vi "AS7261_colorimeter.vi"() -> ()   [LabVIEW 2011]
uses:
  <vilib>/Utility/miscctls.llb/LVAnnotationListTypeDef.ctl
  <vilib>/Instr/_visa.llb/VISA Configure Serial Port (Instr).vi
  <vilib>/Analysis/baseanly.llb/A x Vector.vi
  <vilib>/Utility/file.llb/Write To Spreadsheet File (DBL).vi
  <vilib>/Analysis/NI_AALBase.lvlib
panel:
  in  "chrm. adaptation":bool
  in  "OK Button 3":bool
  in  "OK Button 2":bool
  out "count":u16
  out "CTN":string
  out "xy":string
  out "RGB":string
  out "XYZ data":string
  out "XYZ array":dbl[](array[numeric])
  in  "CWDataServer.ICWDataServer":refnum<k7>
  in  "OK Button":bool
  in  "correction":string(combo)="to gamma RGB"
  out "Color Box 3":u32(colorbox)
  in  "Radio Buttons":enum32{"Radio Selection 1", "Radio Selection 2"}(radio)
  in  "sRGB 5":bool
  in  "sRGB 4":bool
  in  "DATA":string(combo)="ATDATA"
  in  "LED1 current":string(combo)="0"
  in  "LED0 current":string(combo)="0"
  in  "sRGB 3":bool
  in  "sRGB 2":bool
  in  "sRGB":bool
  in  "Gain":string(combo)="2"
  in  "Integration time [ms]":dbl(slide)=198.79999999999998 min=2.8 max=714.0 step=2.8 scale=2.8..714.0
  in  "stop":bool
  in  "COM port":refnum<visa-resource-name>
  out "CIE 1931":cluster{dbl[], dbl[]}[](graph)=[{[nan], [nan]}, {[], []}, {[], []}, {[], []}, {[], []}, {[], []}]
  # "RGB color space"
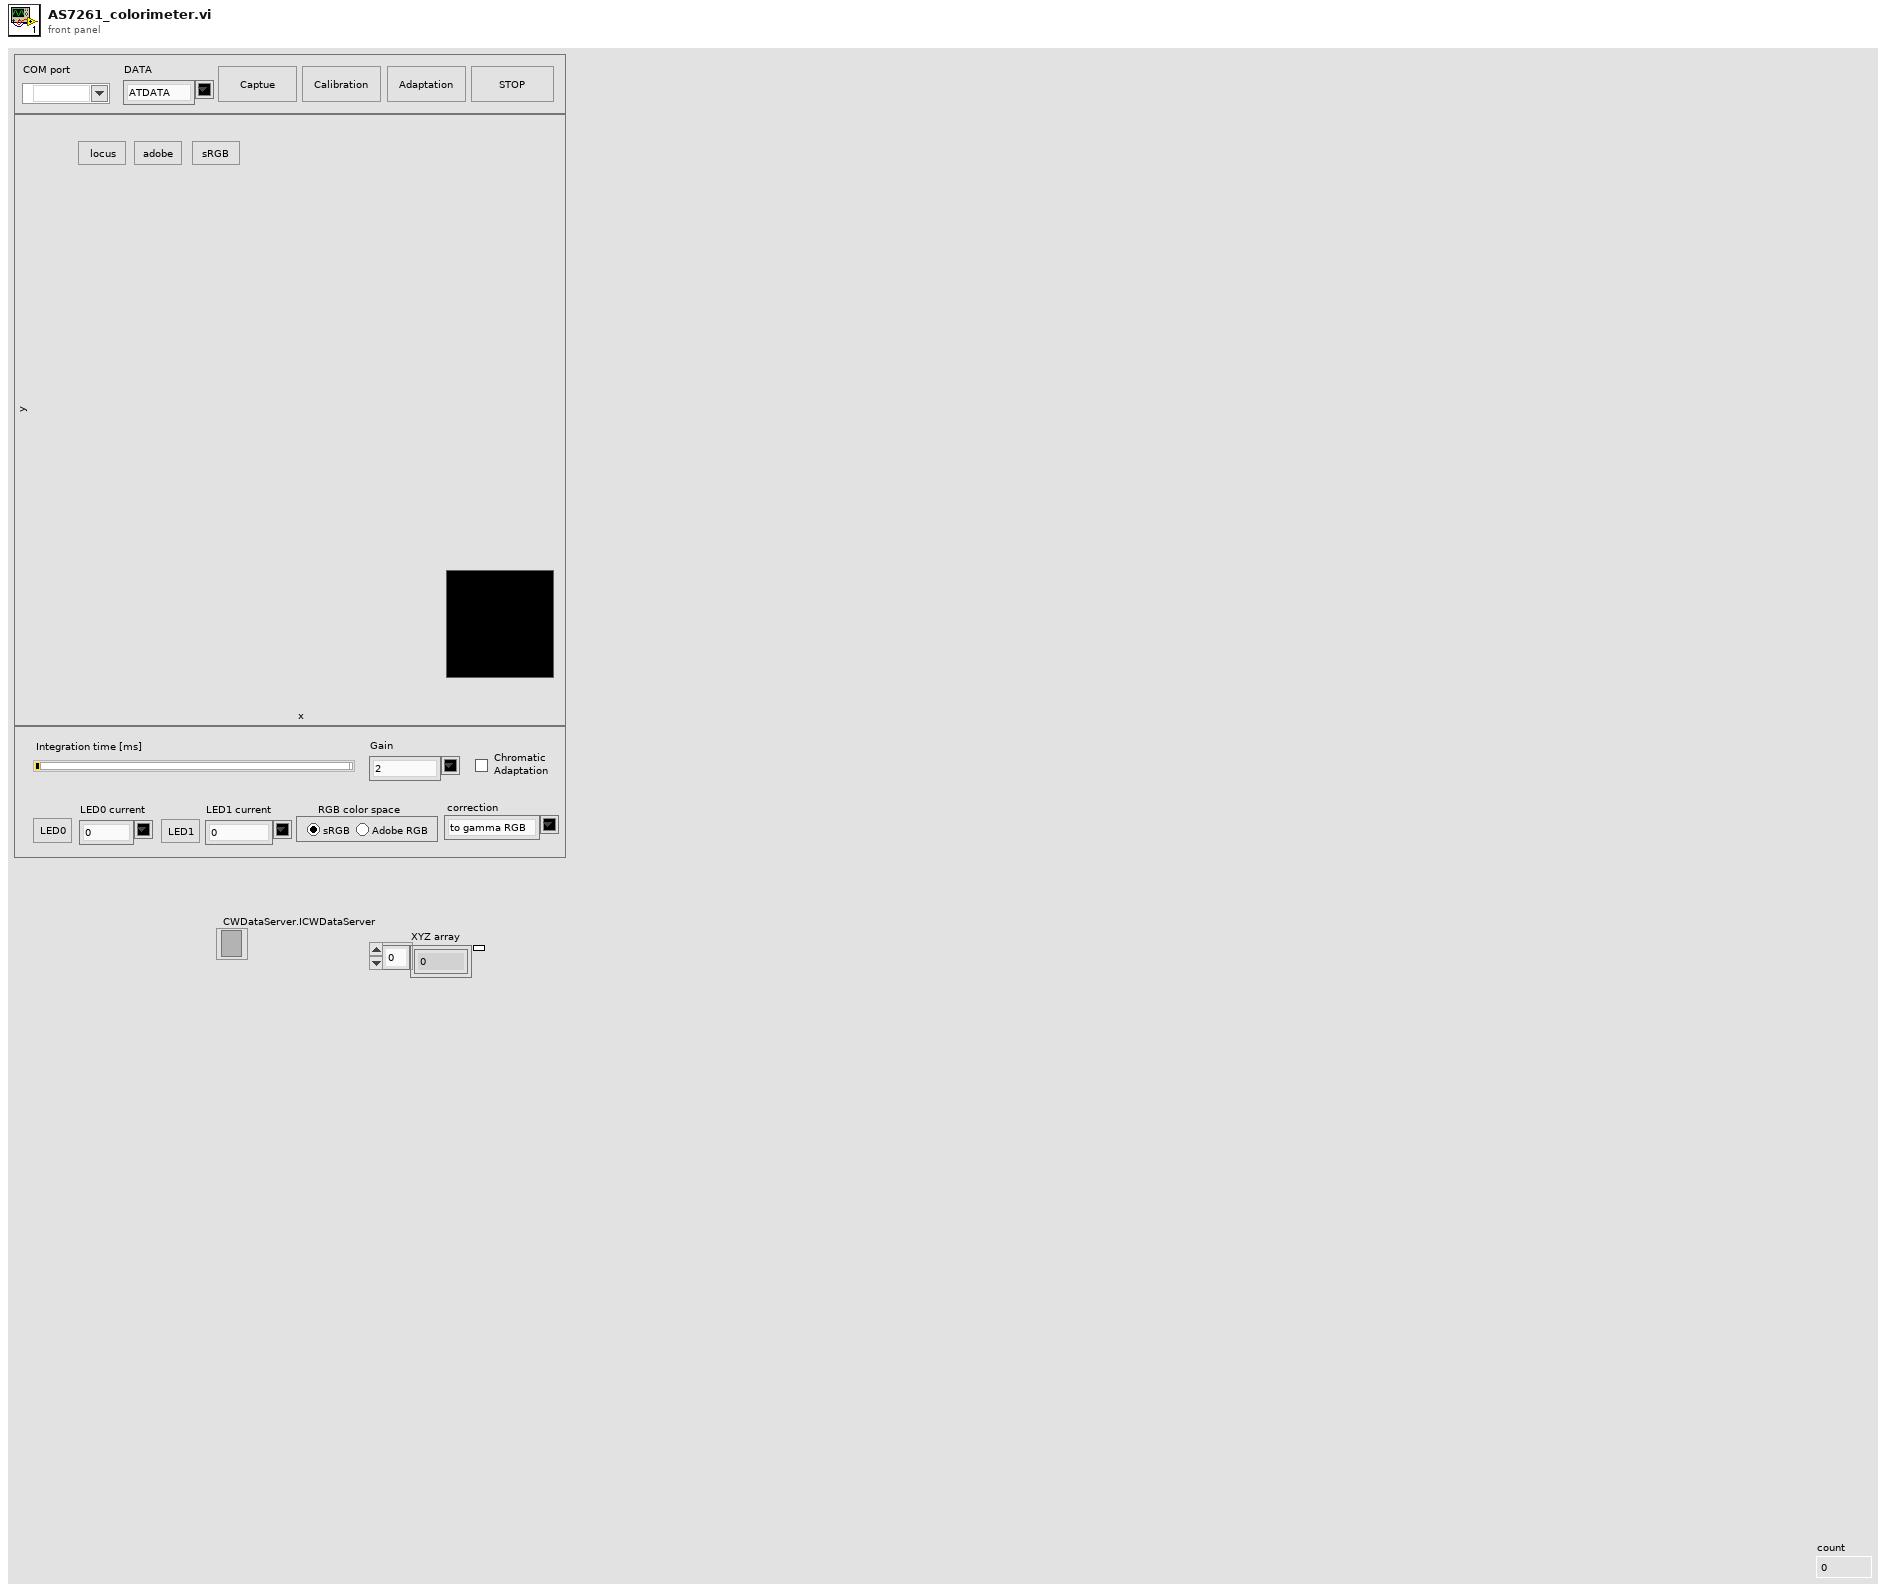
[diagram p1: front panel]
types:
  T1 = typedef "LVRangeTypeDef.ctl" = cluster{"Minimum":dbl, "Maximum":dbl, "Increment":dbl, "Minor Increment":dbl, "Start":dbl}
  T2 = typedef "LVBoundsTypeDef.ctl" = cluster{"Width":u32, "Height":u32}
  T3 = typedef "NI_Matrix.lvlib/RealMatrix.ctl" = dbl[][]
  T4 = enum32{"Invalid", "Standard", "Closed", "Hidden", "Minimized", "Maximized"}
  T5 = typedef "LVAnnotationListTypeDef.ctl" = cluster{"Name":string, "Color":u32, "Style":u8, "Point Style":u8, "Name Visible":bool, "Allow Drag":bool, "Annotation Mode":u32, "Plot":i32, "Index":i32, "Position":cluster{"X":dbl, "Y":dbl}, "X Scale":u32, "Y Scale":u32, "Show Arrow":bool, "Lock Name":bool, "Plot Area":i32, "Label Offset":cluster{"X":dbl, "Y":dbl}}[]
  T6 = cluster{"Name":string, "Color":u32, "Style":u8, "Point Style":u8, "Name Visible":bool, "Allow Drag":bool, "Annotation Mode":u32, "Plot":i32, "Index":i32, "Position":cluster{"X":dbl, "Y":dbl}, "X Scale":u32, "Y Scale":u32, "Show Arrow":bool, "Lock Name":bool, "Plot Area":i32, "Label Offset":cluster{"X":dbl, "Y":dbl}}[]
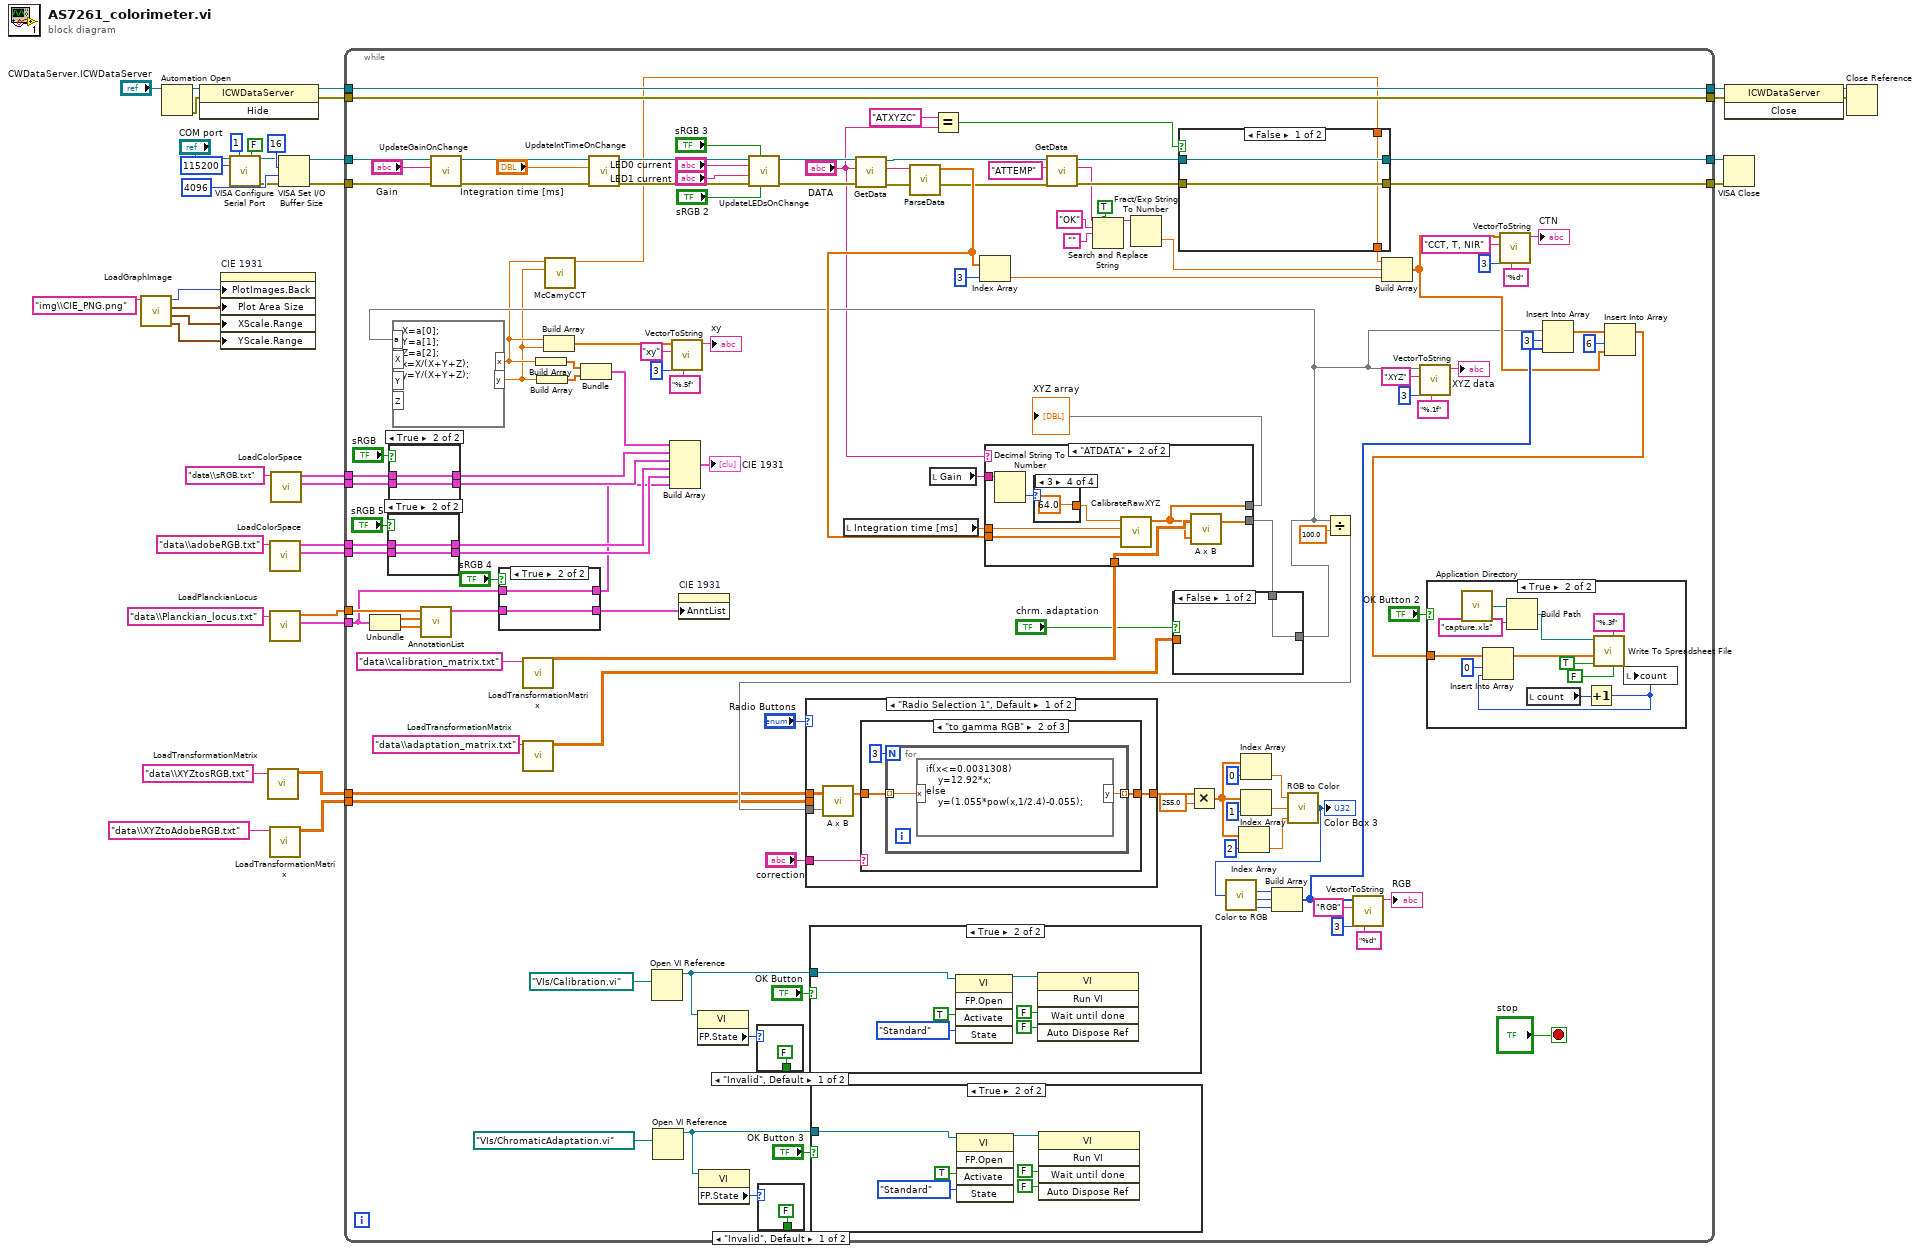
[diagram p0: block diagram]
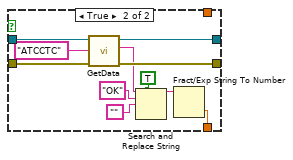
[diagram p2: hidden frame]
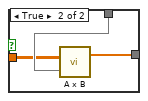
[diagram p3: hidden frame]
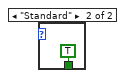
[diagram p4: hidden frame]
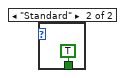
[diagram p7: hidden frame]
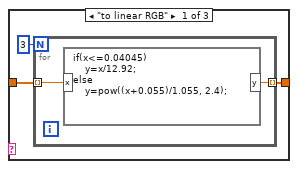
[diagram p9: hidden frame]
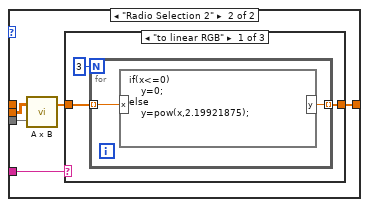
[diagram p11: hidden frame]
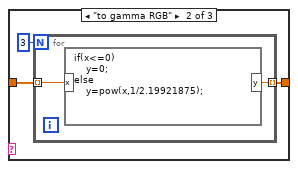
[diagram p12: hidden frame]
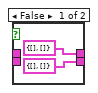
[diagram p14: hidden frame]
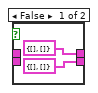
[diagram p15: hidden frame]
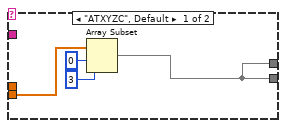
[diagram p16: hidden frame]
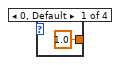
[diagram p17: hidden frame]
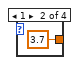
[diagram p18: hidden frame]
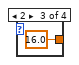
[diagram p19: hidden frame]
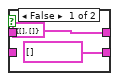
[diagram p20: hidden frame]
diagram:
  n1 = call "LoadGraphImage.vi"("relative path"="img\\CIE_PNG.png" ("name or relative path")) -> ("Y Scale.Range"=w12:T1, "X Scale.Range"=w13:T1, "PlotAreaSize"=w14:T2, "picture"=w1:picture)  [unwired: 7 in]
  n2 = Automation Open(Automation Refnum="CWDataServer.ICWDataServer") -> (Automation Refnum=w8:refnum<k7>, error out=w9:errorcluster)  [unwired: 3 in]
  n3 = invoke class="ICWDataServer" method="Hide"(reference=w8, error in=w9) -> (reference out=w7:refnum<k7>, error out=w6:errorcluster)  [unwired: 1 in, 1 out]
  n4 = property on="CIE 1931" class="XYGraph (strict)"("PlotImages.Back"=w1, "Plot Area Size"=w14, "XScale.Range"=w13, "YScale.Range"=w12) -> ()  [unwired: 2 in, 2 out]
  n5 = call-poly "VISA Configure Serial Port"("VISA resource name"="COM port", "timeout (10sec)"=u32 1, "Enable Termination\nChar (T)"=FALSE ("Enable Termination\nChar (T)"), "baud rate (9600)"=u32 115200) -> ("VISA resource name out"=w32:refnum<visa-resource-name>, "error out"=w31:errorcluster)  [unwired: 10 in]
  n6 = call "LoadTransformationMatrix.vi"("relative path"="data\\XYZtosRGB.txt" ("name or relative path")) -> ("transformation matrix"=w16:T3)  [unwired: 10 in]
  n7 = call "LoadColorSpace.vi"("relative path"="data\\adobeRGB.txt" ("name or relative path")) -> ("white"=w22:cluster{dbl[], dbl[]}, "gamut"=w23:cluster{dbl[], dbl[]})  [unwired: 9 in]
  n8 = call "LoadPlanckianLocus.vi"("relative path"="data\\Planckian_locus.txt" ("name or relative path")) -> ("Planckian locus"=w18:cluster{"all rows":dbl[], "all rows":dbl[]}, "CCTs"=w17:dbl[])  [unwired: 9 in]
  n9 = call "LoadTransformationMatrix.vi"("relative path"="data\\XYZtoAdobeRGB.txt" ("name or relative path")) -> ("transformation matrix"=w15:T3)  [unwired: 10 in]
  n10 = call "LoadColorSpace.vi"("relative path"="data\\sRGB.txt" ("name or relative path")) -> ("white"=w25:cluster{dbl[], dbl[]}, "gamut"=w24:cluster{dbl[], dbl[]})  [unwired: 9 in]
  n11 = VISA Set I/O Buffer Size(VISA resource name=w32, mask (16)=u16 16 ("I/O Receive\nBuffer mask"), size (4096)=u32 4096, error in (no error)=w31) -> (VISA resource name out=w35:refnum<visa-resource-name>, error out=w36:errorcluster)
  n12 = while {
    tunnel: w36 -> [w82]
    tunnel: w35 -> [w83]
    tunnel: [w64] -> w38
    tunnel: [w63] -> w37
    tunnel: w25 -> [w151]
    tunnel: w24 -> [w150]
    tunnel: w23 -> [w147]
    tunnel: w22 -> [w148]
    tunnel: w18 -> [w138]
    tunnel: w17 -> [w143]
    tunnel: w16 -> [w119]
    tunnel: w15 -> [w120]
    tunnel: w7 -> [w114]
    tunnel: [w114] -> w3
    tunnel: w6 -> [w113]
    tunnel: [w113] -> w2
    stop <- "stop" stop-if-true
    n13 = Unbundle(w138) -> ("all rows"=w145:dbl[], "all rows"=w144:dbl[])
    n14 = case shown="True" "sRGB 5" {
      tunnel: w148 -> [_ w244]
      tunnel: [cluster{dbl[], dbl[]} {[], []} ("white") w244] -> w139
      tunnel: w147 -> [_ w243]
      tunnel: [cluster{dbl[], dbl[]} {[], []} ("gamut") w243] -> w140
      frame False {
      }
      frame True {
      }
    }
    n15 = case shown="True" "sRGB" {
      tunnel: w151 -> [_ w248]
      tunnel: [cluster{dbl[], dbl[]} {[], []} ("white") w248] -> w141
      tunnel: w150 -> [_ w247]
      tunnel: [cluster{dbl[], dbl[]} {[], []} ("gamut") w247] -> w142
      frame False {
      }
      frame True {
      }
    }
    n16 = call "AnnotationList.vi"("y array"=w144, "x array"=w145, "annotations"=w143) -> ("annotation list"=w135:T6)  [unwired: 8 in]
    n17 = call "UpdateGainOnChange.vi"("error in"=w82, "Gain"="Gain", "VISA resource name in"=w83) -> ("error out"=w80:errorcluster, "VISA resource name out"=w81:refnum<visa-resource-name>)  [unwired: 7 in]
    n18 = case shown="True" "sRGB 4" {
      tunnel: [cluster{dbl[], dbl[]} {[], []} w268] -> w136
      tunnel: w138 -> [_ w268]
      tunnel: w135 -> [_ w267]
      tunnel: [T5 [] ("Annotation List") w267] -> w134
      frame False {
      }
      frame True {
      }
    }
    n19 = call "LoadTransformationMatrix.vi"("relative path"="data\\calibration_matrix.txt" ("name or relative path")) -> ("transformation matrix"=w110:T3)  [unwired: 10 in]
    n20 = call "LoadTransformationMatrix.vi"("relative path"="data\\adaptation_matrix.txt" ("name or relative path")) -> ("transformation matrix"=w48:T3)  [unwired: 10 in]
    n21 = call "UpdateIntTimeOnChange.vi"("error in"=w80, "Integration time [ms]"="Integration time [ms]", "VISA resource name in"=w81) -> ("error out"=w77:errorcluster, "VISA resource name out"=w78:refnum<visa-resource-name>)  [unwired: 7 in]
    n22 = Open VI Reference(vi path=path "VIs/Calibration.vi") -> (vi reference=w117:refnum<vi>)  [unwired: 5 in, 1 out]
    n23 = Open VI Reference(vi path=path "VIs/ChromaticAdaptation.vi") -> (vi reference=w53:refnum<vi>)  [unwired: 5 in, 1 out]
    n24 = property on="CIE 1931" class="XYGraph (strict)"("AnntList"=w134) -> ()  [unwired: 2 in, 2 out]
    n25 = property class="VI"(reference=w117) -> ("FP.State"=w116:T4)  [unwired: 1 in, 2 out]
    n26 = property class="VI"(reference=w53) -> ("FP.State"=w52:T4)  [unwired: 1 in, 2 out]
    n27 = call "UpdateLEDsOnChange.vi"("LED1"="sRGB 2", "LED0"="sRGB 3", "error in"=w77, "LED1 current"="LED1 current", "LED0 current"="LED0 current", "VISA resource name in"=w78) -> ("error out"=w71:errorcluster, "VISA resource name out"=w72:refnum<visa-resource-name>)  [unwired: 4 in]
    n28 = case shown="\"Invalid\", Default" w116 {
      tunnel: [FALSE TRUE] -> _
      frame "Invalid", Default {
      }
      frame "Standard" {
      }
    }
    n29 = case shown="\"Invalid\", Default" w52 {
      tunnel: [FALSE TRUE] -> _
      frame "Invalid", Default {
      }
      frame "Standard" {
      }
    }
    n30 = case shown="True" "OK Button" {
      tunnel: w117 -> [_ w206]
      frame False {
      }
      frame True {
        n31 = invoke class="VI" method="FP.Open"(reference=w206, "Activate"=TRUE ("Activate?"), "State"=T4."Standard") -> (reference out=w205:refnum<vi>)  [unwired: 2 in, 4 out]
        n32 = invoke class="VI" method="Run VI"(reference=w205, "Wait until done"=FALSE ("Wait Until Done"), "Auto Dispose Ref"=FALSE ("Auto Dispose Reference")) -> ()  [unwired: 2 in, 5 out]
      }
    }
    n33 = case shown="True" "OK Button 3" {
      tunnel: w53 -> [_ w187]
      frame False {
      }
      frame True {
        n34 = invoke class="VI" method="FP.Open"(reference=w187, "Activate"=TRUE ("Activate?"), "State"=T4."Standard") -> (reference out=w186:refnum<vi>)  [unwired: 2 in, 4 out]
        n35 = invoke class="VI" method="Run VI"(reference=w186, "Wait until done"=FALSE ("Wait Until Done"), "Auto Dispose Ref"=FALSE ("Auto Dispose Reference")) -> ()  [unwired: 2 in, 5 out]
      }
    }
    n36 = local read "Integration time [ms]"() -> (w152:dbl)
    n37 = call "GetData.vi"("error in (no error)"=w71, "DATA"="DATA", "VISA Refnum in"=w72) -> ("error out"=w68:errorcluster, "data"=w70:string, "VISA Refnum out"=w69:refnum<visa-resource-name>)  [unwired: 6 in]
    n38 = call "ParseData.vi"("DATA"=w70) -> ("data"=w109:dbl[])  [unwired: 10 in]
    n39 = local read "Gain"() -> (w133:string)
    n40 = Equal?(x="ATXYZC", y="DATA") -> (x = y?=w41:bool)
    n41 = Index Array(array=w109, index=3) -> (element=w85:dbl)
    n42 = case shown="\"ATDATA\"" "DATA" {
      tunnel: w109 -> [w252 w260]
      tunnel: [w249 w254] -> w47
      tunnel: w152 -> [_ w259]
      tunnel: w133 -> [_ w256]
      tunnel: w110 -> [_ w255]
      tunnel: [w249 w253] -> w112
      frame "ATXYZC", Default {
        n43 = Array Subset(array=w252, index=0, length=3) -> (w249:dbl[])
      }
      frame "ATDATA" {
        n44 = Decimal String To Number(string=w256) -> (number=w258:i32)  [unwired: 2 in, 1 out]
        n45 = case shown="3" w258 {
          tunnel: [1.0 ("Label Offset.X") 3.7 ("Label Offset.X") 16.0 ("Label Offset.X") 64.0 ("Label Offset.X")] -> w257
          frame 0, Default {
          }
          frame 1 {
          }
          frame 2 {
          }
          frame 3 {
          }
        }
        n46 = call "CalibrateRawXYZ.vi"("raw XYZ array"=w260, "integration time"=w259, "gain"=w257) -> ("XYZ array"=w253:dbl[])  [unwired: 8 in]
        n47 = call-poly <vilib>:"A x B.vi"("Vector"=w253, "A"=w255) -> ("A x Vector"=w254:dbl[])  [unwired: 1 out]
      }
    }
    "XYZ array" <- w112
    n48 = call "GetData.vi"("error in (no error)"=w68, "DATA"="ATTEMP" ("string"), "VISA Refnum in"=w69) -> ("error out"=w66:errorcluster, "data"=w62:string, "VISA Refnum out"=w67:refnum<visa-resource-name>)  [unwired: 6 in]
    n49 = Search and Replace String(replace all?=TRUE ("replace all? (F)"), input string=w62, search string="OK" ("substring (\"\")"), replace string="") -> (result string=w154:string)  [unwired: 4 in, 3 out]
    n50 = Fract/Exp String To Number(string=w154) -> (number=w86:dbl)  [unwired: 3 in, 1 out]
    n51 = case shown="False" "chrm. adaptation" {
      tunnel: w48 -> [_ w180]
      tunnel: w47 -> [w178 w181]
      tunnel: [w178 w179] -> w46
      frame False {
      }
      frame True {
        n52 = call-poly <vilib>:"A x B.vi"("Vector"=w181, "A"=w180) -> ("A x Vector"=w179:dbl[])  [unwired: 1 out]
      }
    }
    n53 = formula code="X=a[0];\nY=a[1];\nZ=a[2];\nx=X/(X+Y+Z);\ny=Y/(X+Y+Z);"("a"=w46) -> ("x"=w45:dbl, "y"=w44:dbl)  [unwired: 3 out]
    n54 = Build Array(w45) -> (w161:dbl[])
    n55 = Build Array(w44) -> (w160:dbl[])
    n56 = Build Array(w45, w44) -> (w92:dbl[])
    n57 = call "McCamyCCT.vi"("y"=w44, "x"=w45) -> ("CCT"=w40:dbl)  [unwired: 9 in]
    n58 = Bundle(w161, w160) -> (w159:cluster{dbl[], dbl[]})  [unwired: 1 in]
    n59 = Build Array(w159, w142, w141, w140, w139, w136) -> (→"CIE 1931":cluster{"all rows":dbl[], "all rows":dbl[]}[])
    n60 = call "VectorToString.vi"("format"="%.5f", "vector length"=3, "name"="xy", "vector"=w92) -> ("string"=→"xy":string)  [unwired: 7 in]
    n61 = case shown="False" w41 {
      tunnel: [w164 w173] -> w87
      tunnel: w67 -> [w166 w172]
      tunnel: w66 -> [w165 w171]
      tunnel: [w166 w169] -> w64
      tunnel: [w165 w168] -> w63
      tunnel: w40 -> [w164 _]
      frame False {
      }
      frame True {
        n62 = call "GetData.vi"("error in (no error)"=w171, "DATA"="ATCCTC" ("string"), "VISA Refnum in"=w172) -> ("error out"=w168:errorcluster, "data"=w167:string, "VISA Refnum out"=w169:refnum<visa-resource-name>)  [unwired: 6 in]
        n63 = Search and Replace String(replace all?=TRUE ("replace all? (F)"), input string=w167, search string="OK" ("substring (\"\")"), replace string="") -> (result string=w174:string)  [unwired: 4 in, 3 out]
        n64 = Fract/Exp String To Number(string=w174) -> (number=w173:dbl)  [unwired: 3 in, 1 out]
      }
    }
    n65 = Divide(x=w46, y=100.0 ("Label Offset.Y")) -> (x/y=w123:dbl[])
    n66 = case shown="\"Radio Selection 1\", Default" "Radio Buttons" {
      tunnel: w119 -> [w213 _]
      tunnel: w123 -> [w212 w228]
      tunnel: "correction" -> [w211 w227]
      tunnel: [w210 w226] -> w121
      tunnel: w120 -> [_ w225]
      frame "Radio Selection 1", Default {
        n67 = call-poly <vilib>:"A x B.vi"("Vector"=w212, "A"=w213) -> ("A x Vector"=w209:dbl[])  [unwired: 1 out]
        n68 = case shown="\"to gamma RGB\"" w211 {
          tunnel: [w214 w219 w224] -> w210
          tunnel: w209 -> [w215 w220 w224]
          frame "to linear RGB" {
            n69 = for {
              N: 3 -> [_]
              tunnel: w215 -> [w218] mode=indexing
              tunnel: [w217] -> w214 mode=indexing
              n70 = formula code="if(x<=0.04045)\n    y=x/12.92;\nelse\n    y=pow((x+0.055)/1.055, 2.4);"("x"=w218) -> ("y"=w217:dbl)
            }
          }
          frame "to gamma RGB" {
            n71 = for {
              N: 3 -> [_]
              tunnel: w220 -> [w222] mode=indexing
              tunnel: [w223] -> w219 mode=indexing
              n72 = formula code="if(x<=0.0031308)\n    y=12.92*x;\nelse\n    y=(1.055*pow(x,1/2.4)-0.055);"("x"=w222) -> ("y"=w223:dbl)
            }
          }
          frame "none", Default {
          }
        }
      }
      frame "Radio Selection 2" {
        n73 = call-poly <vilib>:"A x B.vi"("Vector"=w228, "A"=w225) -> ("A x Vector"=w229:dbl[])  [unwired: 1 out]
        n74 = case shown="\"to linear RGB\"" w227 {
          tunnel: [w230 w235 w240] -> w226
          tunnel: w229 -> [w231 w236 w240]
          frame "to linear RGB" {
            n75 = for {
              N: 3 -> [_]
              tunnel: w231 -> [w234] mode=indexing
              tunnel: [w233] -> w230 mode=indexing
              n76 = formula code="if(x<=0)\n    y=0;\nelse\n    y=pow(x,2.19921875);"("x"=w234) -> ("y"=w233:dbl)
            }
          }
          frame "to gamma RGB" {
            n77 = for {
              N: 3 -> [_]
              tunnel: w236 -> [w238] mode=indexing
              tunnel: [w239] -> w235 mode=indexing
              n78 = formula code="if(x<=0)\n    y=0;\nelse\n    y=pow(x,1/2.19921875);"("x"=w238) -> ("y"=w239:dbl)
            }
          }
          frame "none", Default {
          }
        }
      }
    }
    n79 = Multiply ("Multiply.vi")(x=w121, y=255.0 ("Label Offset.Y")) -> (x*y=w126:dbl[])
    n80 = Index Array(array=w126, index=2) -> (element=w127:dbl)
    n81 = Index Array(array=w126, index=0) -> (element=w128:dbl)
    n82 = Index Array(array=w126, index=1) -> (element=w125:dbl)
    n83 = call <vilib>:"RGB to Color.vi"("B"=w127, "G"=w125, "R"=w128) -> ("Color"=w101:u32)
    "Color Box 3" <- w101
    n84 = call <vilib>:"Color to RGB.vi"("Color"=w101) -> ("R"=w104:u8, "G"=w103:u8, "B"=w102:u8)  [unwired: 1 out]
    n85 = Build Array(w104, w103, w102) -> (w60:u8[])
    n86 = call "VectorToString.vi"("format"="%d", "vector length"=3, "name"="RGB", "vector"=w60) -> ("string"=→"RGB":string)  [unwired: 7 in]
    n87 = Build Array(w87, w86, w85) -> (w57:dbl[])
    n88 = call "VectorToString.vi"("format"="%.1f", "vector length"=3, "name"="XYZ", "vector"=w46) -> ("string"=→"XYZ data":string)  [unwired: 7 in]
    n89 = call "VectorToString.vi"("format"="%d", "vector length"=3, "name"="CCT, T, NIR", "vector"=w57) -> ("string"=→"CTN":string)  [unwired: 7 in]
    n90 = Insert Into Array(array=w46, index=3, new element=w60) -> (w58:dbl[])
    n91 = Insert Into Array(array=w58, index=6, new element=w57) -> (w55:dbl[])
    n92 = case shown="True" "OK Button 2" {
      tunnel: w55 -> [_ w190]
      frame False {
      }
      frame True {
        n93 = call <vilib>:"Application Directory.vi"() -> ("Application Directory"=w193:path)
        n94 = Build Path(base path=w193, name or relative path="capture.xls") -> (appended path=w191:path)
        n95 = local read "count"() -> (w197:u16)
        n96 = Increment(x=w197) -> (x+1=w195:u16)
        n97 = Insert Into Array(array=w190, index=0, new element=w195) -> (w194:dbl[])
        n98 = call-poly <vilib>:"Write To Spreadsheet File.vi"("transpose? (no:F)"=FALSE, "format (%.3f)"="%.3f", "append to file? (new file:F)"=TRUE, "1D data"=w194, "file path (dialog if empty)"=w191) -> ()  [unwired: 3 in, 1 out]
        n99 = local write "count"(w195) -> ()
      }
    }
  }
  n100 = VISA Close(VISA resource name=w38, error in (no error)=w37) -> ()  [unwired: 1 out]
  n101 = invoke class="ICWDataServer" method="Close"(reference=w3, error in=w2) -> (reference out=w5:refnum<k7>, error out=w4:errorcluster)  [unwired: 1 in, 1 out]
  n102 = Close Reference(reference=w5, error in (no error)=w4) -> ()  [unwired: 1 out]
